vi "ContinuousShow1.vi"() -> ()   [LabVIEW 2017]
uses:
  <vilib>/express/express analysis/Spectral/Block/exnSpectralBlock spectral measurements RMS poly.vi
  <vilib>/express/express analysis/Spectral/Block/exnSpectralBlock spectral measurements RMS DDT.vi
  <vilib>/express/express analysis/Spectral/XNode/ExpressSpectralMeasurementsBlockNode.xnode
panel:
  out "Power":dbl
  out "Waveform Chart 2":dynamicdata(graph)
  out "Waveform Chart 4":dynamicdata(graph)
  out "Waveform Chart":dynamicdata(graph)
  out "Waveform Chart 3":dynamicdata(graph)
  in  "stop (F)":bool
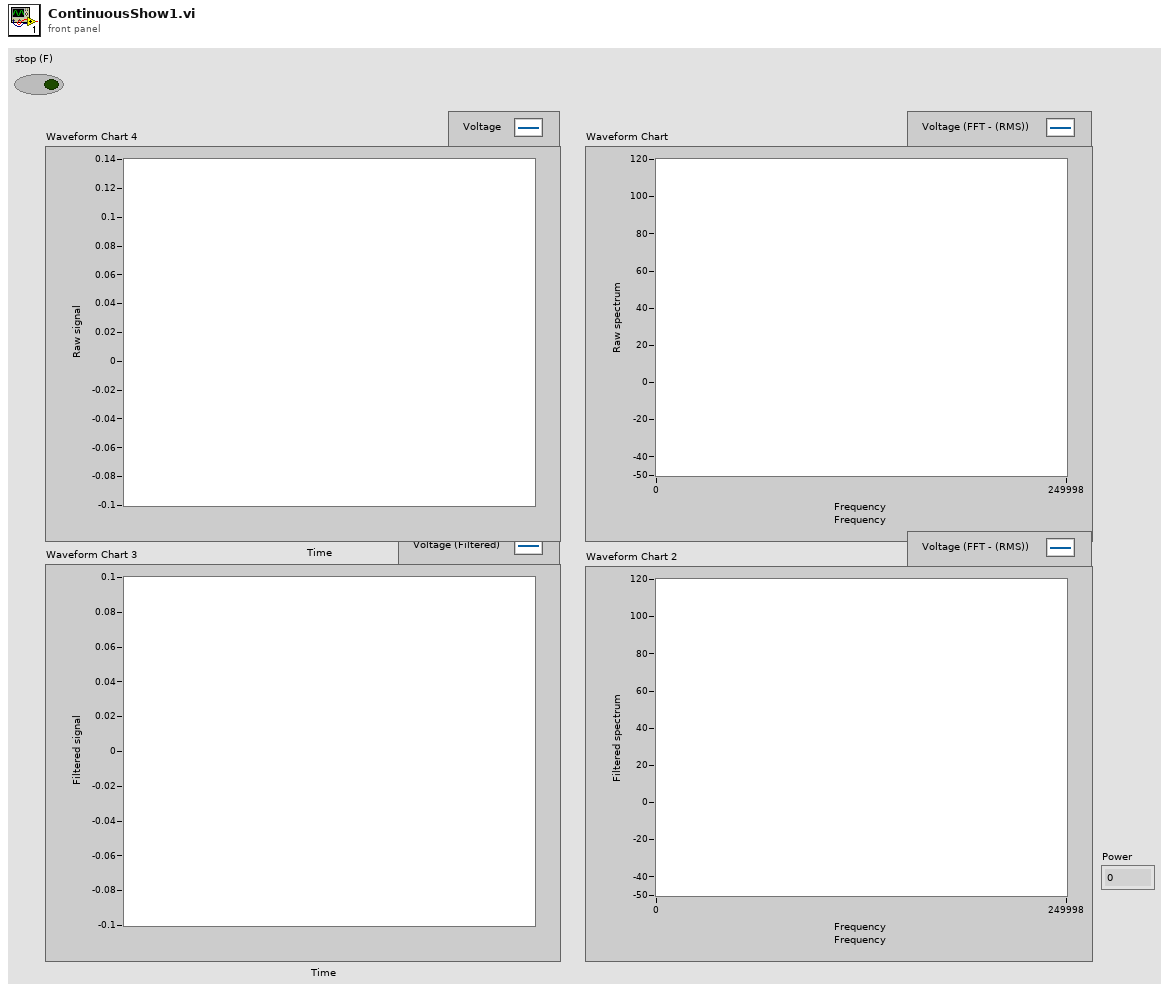
[diagram p1: front panel]
types:
  T1 = cluster{"averaging mode":u16, "weighting mode":u16, "number of averages":u32}
  T2 = cluster{"dB On (F)":bool, "unwrap phase (F)":bool, "convert to degree (F)":bool}
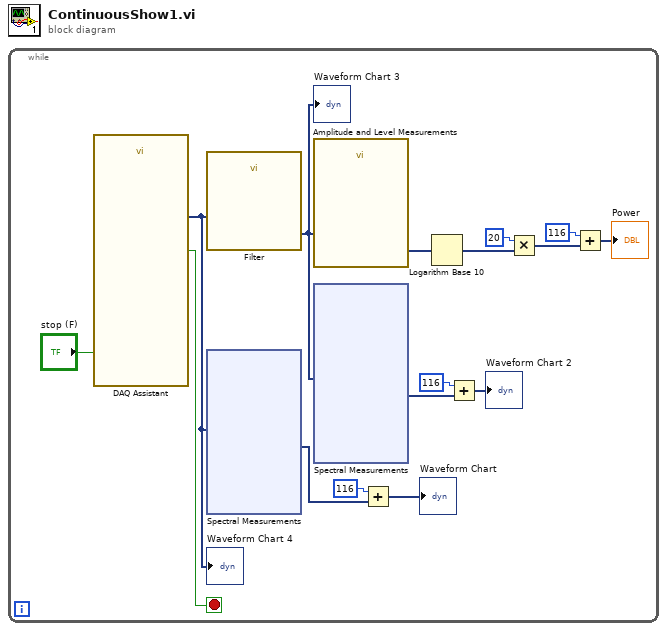
[diagram p0: block diagram]
diagram:
  n1 = while {
    stop <- w16 stop-if-true
    n2 = call "DAQ Assistant"("stop (F)"="stop (F)") -> ("data"=w14:dynamicdata, "stopped"=w16:bool)  [unwired: 15 in, 2 out]
    "Waveform Chart 4" <- w14
    n3 = call "Filter"("Signal"=w14) -> ("Filtered Signal"=w7:dynamicdata)  [unwired: 9 in, 1 out]
    "Waveform Chart 3" <- w7
    n4 = xnode "Spectral Measurements"("Signals"=w14) -> ("FFT - (RMS)"=w13:dynamicdata)  [unwired: 1 in, 2 out]
    n5 = call "Amplitude and Level Measurements"("Signals"=w7) -> ("RMS"=w5:dynamicdata)  [unwired: 13 in, 1 out]
    n6 = xnode "Spectral Measurements"("Signals"=w7) -> ("FFT - (RMS)"=w9:dynamicdata)  [unwired: 1 in, 2 out]
    n7 = Add(x=116, y=w13) -> (x+y=→"Waveform Chart":dynamicdata)
    n8 = Logarithm Base 10(1:w5) -> (0:w4:dynamicdata)
    n9 = Add(x=116, y=w9) -> (x+y=→"Waveform Chart 2":dynamicdata)
    n10 = Multiply(x=20, y=w4) -> (x*y=w3:dynamicdata)
    n11 = Add(x=116, y=w3) -> (x+y=→"Power":dynamicdata)
  }
